vi "ROI grp-Save Load Groups header.vi"(8 "error in (no error)":errorcluster, 9 "POI groups header file data (in)":string[][](array[string]), 11 "Function":T1=enum."Load file") -> (0 "error out":errorcluster, 1 "POI groups header file data":string[][](array[string]), 3 "POI groups column header":string[](array[string]))   [LabVIEW 2020]
uses:
  Experiment header interface/Typedefs/Save-Load-Save as-Load last enum.ctl
  Global variables/gl_Functional Imaging-Global variables.vi
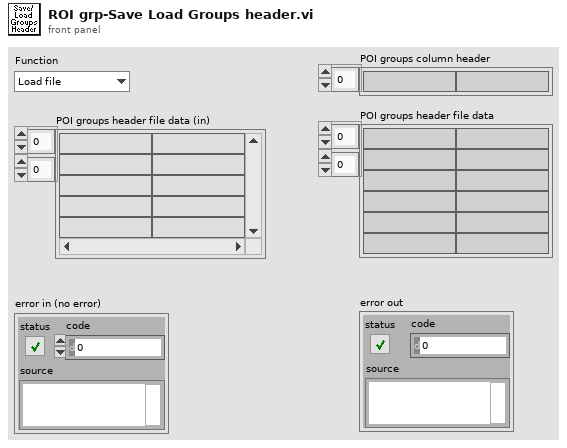
[diagram p1: front panel]
types:
  T1 = typedef "Save-Load-Save as-Load last enum.ctl" = enum16{"Save file", "Save file as", "Load file", "Load last file"}
  T2 = typedef "Functional Imging UI Refs.ctl" = cluster{"Menu ref":refnum<k9>, "Image control":refnum<vi>, "VI ref":refnum<vi>, "XGrapher":refnum<vi>, "Smoothing":refnum<vi>, "POI Averaging":refnum<vi>, "Normalize":refnum<vi>, "POI data points in each trial":refnum<vi>, "Channel":refnum<vi>, "Experiment data folder path":refnum<vi>, "[ROI vis]":refnum<vi>, "[Groups] visbl":T3, "Group Name":refnum<vi>, "POI index":refnum<vi>, "Trial No.":refnum<vi>, "Intensity Zoom":refnum<vi>, "Trial Cursor Enabled":refnum<vi>, "Number of Trials (ind 1)":refnum<vi>, "Number of Trials (ind 2)":refnum<vi>, "MiniScans Available":refnum<vi>, "POI Available":refnum<vi>, "Defer graph updates":refnum<vi>, "Waveform selector":refnum<vi>, "#of selected POI":refnum<vi>, "#of selected MiniScans":refnum<vi>, "#of selected groups":refnum<vi>, "Max Z-Projection":refnum<vi>, "Z-Plane Selector":refnum<vi>, "Index of miniscan point to visualise":refnum<vi>, "ROI vis. mode":refnum<vi>, "Total # of points":refnum<vi>, "Index of group clicked on":refnum<vi>, "Pane 1":refnum<vi>, "Pane 2":refnum<vi>, "Pane 3":refnum<vi>, "Pane 4":refnum<vi>, "Pane 5":refnum<vi>, "Pane 6":refnum<vi>, "Deselect all ROI":refnum<vi>, "Deselect all groups":refnum<vi>}
  T3 = typedef "Groups array referecne.ctl" = refnum<vi>
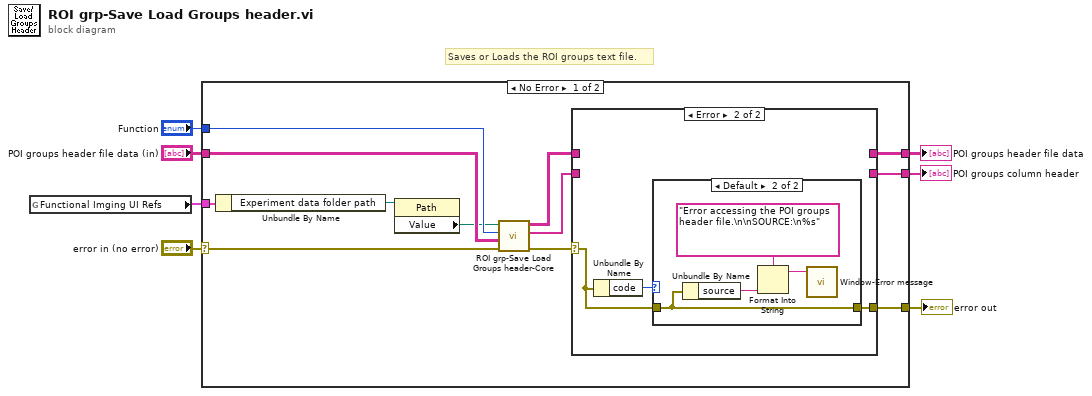
[diagram p0: block diagram]
diagram:
  # "Saves or Loads the ROI groups text file."
  n1 = global read "gl_Functional Imaging-Global variables.vi" "Functional Imging UI Refs"() -> (w1:T2)
  n2 = case shown="No Error" "error in (no error)" {
    selector: "error in (no error)" -> [w14 w29]
    tunnel: "POI groups header file data (in)" -> [w11 _]
    tunnel: "Function" -> [w19 _]
    tunnel: [w15 _] -> w3
    tunnel: [w17 w29] -> w6
    tunnel: [w12 _] -> w2
    tunnel: w1 -> [w8 _]
    frame No Error {
      n3 = Unbundle By Name(w8) -> ("Experiment data folder path"=w10:refnum<vi>)
      n4 = property class="Path"(reference=w10) -> ("Value"=w9:path)  [unwired: 1 in, 2 out]
      n5 = call "ROI grp-Save Load Groups header-Core.vi"("error in (no error)"=w14, "POI groups header file data (& header) to save"=w11, "Function"=w19, "Experiment folder path"=w9) -> ("error out"=w18:errorcluster, "Loaded POI groups header"=w13:string[], "Loaded POI groups table data (No header)"=w16:string[][])  [unwired: 5 in]
      n6 = case shown="Error" w18 {
        selector: w18 -> [_ w24]
        tunnel: [_ w22] -> w17
        tunnel: w16 -> [w21 _]
        tunnel: [w21 _] -> w15
        tunnel: w13 -> [w20 _]
        tunnel: [w20 _] -> w12
        frame No Error {
        }
        frame Error {
          n7 = Unbundle By Name(w24) -> ("code"=w23:i32)
          n8 = case shown="Default" w23 {
            tunnel: w24 -> [_ w25]
            tunnel: [_ w25] -> w22
            frame 7 {
              # "Clears error 7 when a groups setup file does not already exist."
            }
            frame Default {
              n9 = Unbundle By Name(w25) -> ("source"=w27:string)
              n10 = Format Into String(format string="Error accessing the POI groups header file.\n\nSOURCE:\n%s", w27) -> (resulting string=w26:string)  [unwired: 2 in, 1 out]
              n11 = call "Window-Error message.vi"("Message"=w26) -> ()  [unwired: 10 in, 1 out]
            }
          }
        }
      }
    }
    frame Error {
    }
  }
  "error out" <- w6
  "POI groups header file data" <- w3
  "POI groups column header" <- w2
